vi "Resize and Splitter solution.vi"() -> ()   [LabVIEW 2015]
panel:
  in  "Listbox":i32(listbox)
  in  "stop":bool
  out "Waveform Chart":dbl(graph)
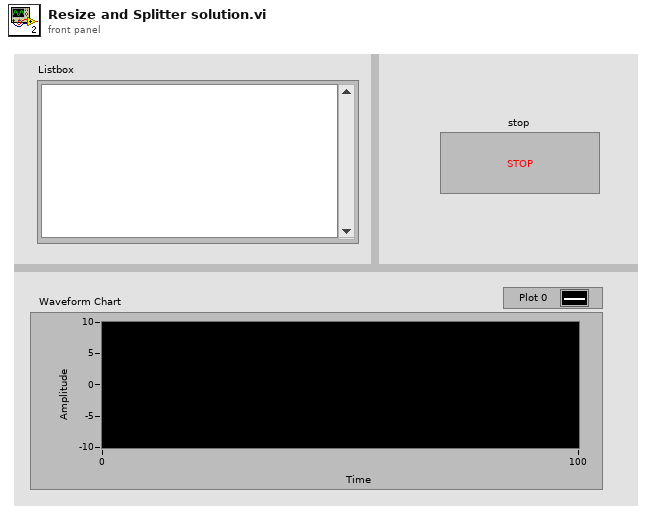
[diagram p1: front panel]
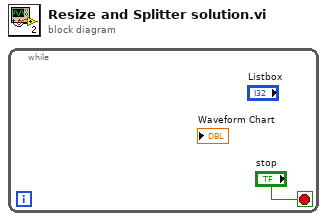
[diagram p0: block diagram]
diagram:
  n1 = while {
    stop <- "stop" stop-if-true
  }
